vi "Inst.KH7008.CreateSMOs.vi"(8 "error in (no error)":errorcluster, 9 "Debug Mode":bool, 11 "Instruments":refnum<class "Inst.Krohn-Hite-7008.lvclass">[](array[class])) -> (0 "error out":errorcluster, 3 "Instruments out":refnum<class "Inst.Krohn-Hite-7008.lvclass">[](array[class]))   [LabVIEW 2019, in "Inst.KH7008.lvlib" / "Inst.Krohn-Hite-7008.lvclass"]
uses:
  Inst.Krohn-Hite-7008.lvclass
  C:/Program Files/National Instruments/LabVIEW 2019/user.lib/LevyLab/Instrument Framework/Instrument/Instrument.lvclass
  <userlib>/LevyLab/Instrument Framework/Instrument/Instrument.lvclass/Instrument.ctl
  Inst.Krohn-Hite-7008.lvclass/Inst.Krohn-Hite-7008.ctl
  <userlib>/LevyLab/Instrument Framework/Instrument/Instrument.lvclass
  <instrlib>/_D2XX/D2XX-LV/D2XX-lv.lvlib
  <instrlib>/_D2XX/D2XX-LV/typedefs/Device Info.ctl
  C:/Program Files/National Instruments/LabVIEW 2019/user.lib/LevyLab/Instrument Framework/Instrument Types/Amplifier/Instrument.Amplifier.lvclass
  C:/Program Files/National Instruments/LabVIEW 2019/vi.lib/JKI/JKI SMO/SMO/SMO.lvclass
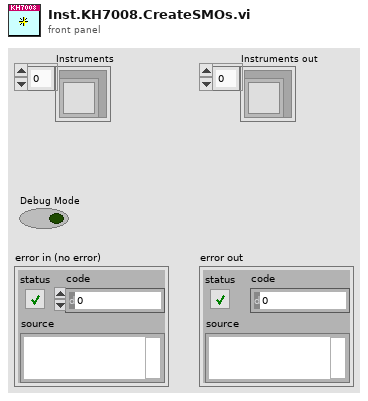
[diagram p1: front panel]
types:
  T1 = typedef "D2XX-lv.lvlib/Device Info.ctl" = cluster{"Serial Number":string, "COM port":string, "Description":string}
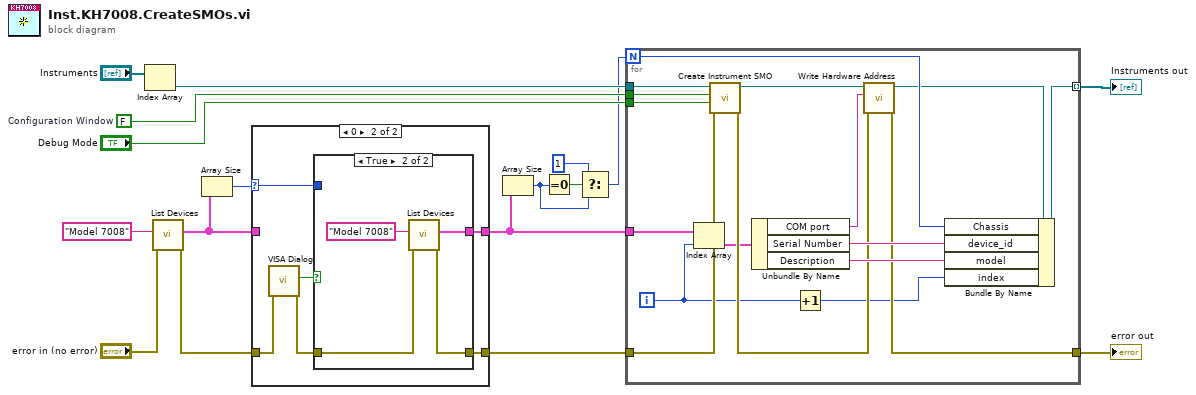
[diagram p0: block diagram]
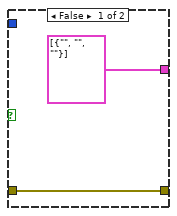
[diagram p3: hidden frame]
diagram:
  w12 = FALSE  # Configuration Window
  n1 = Index Array(array="Instruments") -> (element=w14:refnum<class "Inst.Krohn-Hite-7008.lvclass">)  [unwired: 1 in]
  n2 = call <instrlib>:"List Devices.vi"("error in (no error)"="error in (no error)", "Filter (Device Description)"="Model 7008") -> ("error out"=w6:errorcluster, "Devices"=w4:T1[])  [unwired: 8 in]
  n3 = Array Size(array=w4) -> (size(s)=w5:i32)
  n4 = case shown="0" w5 {
    selector: w5 -> [_ w20]
    tunnel: w6 -> [w19 w25]
    tunnel: [w19 w23] -> w1
    tunnel: w4 -> [w18 _]
    tunnel: [w18 w22] -> w3
    frame Default {
    }
    frame 0 {
      n5 = call "VISA Dialog.vi"("error in"=w25) -> ("error out"=w24:errorcluster, "OK button"=w21:bool)  [unwired: 9 in]
      n6 = case shown="True" w21 {
        tunnel: w24 -> [w26 w30]
        tunnel: [w26 w29] -> w23
        tunnel: [T1[] [{"Serial Number"="", "COM port"="", "Description"=""}] ("Devices") w28] -> w22
        tunnel: w20 -> [_ _]
        frame False {
        }
        frame True {
          n7 = call <instrlib>:"List Devices.vi"("error in (no error)"=w30, "Filter (Device Description)"="Model 7008") -> ("error out"=w29:errorcluster, "Devices"=w28:T1[])  [unwired: 8 in]
        }
      }
    }
  }
  n8 = Array Size(array=w3) -> (size(s)=w2:i32)
  n9 = Equal To 0?(x=w2) -> (x = 0?=w16:bool)
  n10 = Select(t=1, s=w16, f=w2) -> (s? t:f=w7:i32)
  n11 = for {
    N: w7 -> [w39]
    tunnel: w14 -> [w48]
    tunnel: "Debug Mode" -> [w47]
    tunnel: w12 -> [w46]
    tunnel: w1 -> [w45]
    tunnel: [w41] -> w9
    tunnel: w3 -> [w36]
    tunnel: [w33] -> w8 mode=indexing
    i -> [w32]
    n12 = Index Array(array=w36, index=w32) -> (element=w37:T1)
    n13 = call <userlib>:"Create Instrument SMO.vi"("error in (no error)"=w45, "Debug Mode? [F]"=w47, "Configuration Window? [T]"=w46, "Instrument in"=w48) -> ("error out"=w42:errorcluster, "Instrument out"=w35:refnum<class "Inst.Krohn-Hite-7008.lvclass">)  [unwired: 6 in]
    n14 = Unbundle By Name(w37) -> ("COM port"=w40:string, "Serial Number"=w44:string, "Description"=w43:string)
    n15 = Increment(x=w32) -> (x+1=w38:i32)
    n16 = call <userlib>:"Write Hardware Address.vi"("error in (no error)"=w42, "Address"=w40, "Instrument in"=w35) -> ("error out"=w41:errorcluster, "Instrument out"=w34:refnum<class "Inst.Krohn-Hite-7008.lvclass">)  [unwired: 7 in]
    n17 = Bundle By Name(cluster=w34, "Chassis"=w39, "device_id"=w44, "model"=w43, "index"=w38) -> (w33:refnum<class "Inst.Krohn-Hite-7008.lvclass">)
  }
  "Instruments out" <- w8
  "error out" <- w9
